vi "Get Temperature Offset.vi"(8 "error in (no error)":errorcluster, 11 "VISA resource name":refnum<visa-resource-name>) -> (0 "error out":errorcluster, 1 "Temperature Units":i32, 2 "Temperature Offset":dbl format="%.4f", 3 "VISA resource name out":refnum<visa-resource-name>)   [LabVIEW 2013, in "Fluke 5XXX Series Multicalibrators.lvlib"]
doc: "This VI returns the temperature offset used for thermocouple measurements (±500 °C).\n\nNote:\n\nThis VI is available only for instrument models 5500A and 5520A."
uses:
  Fluke 5XXX Series Multicalibrators.lvlib
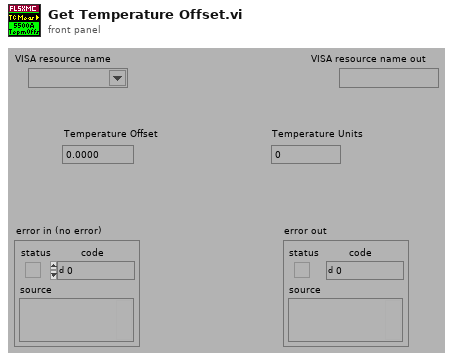
[diagram p1: front panel]
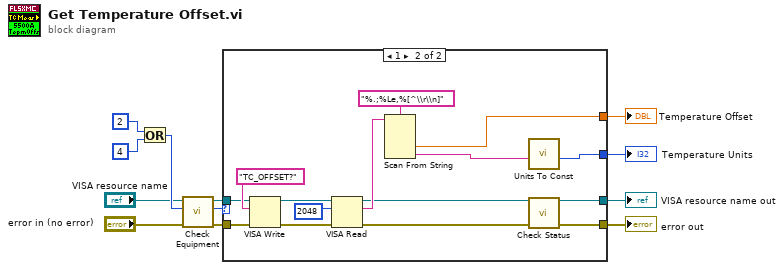
[diagram p0: block diagram]
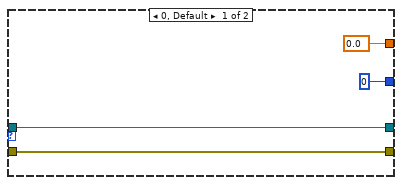
[diagram p2: hidden frame]
diagram:
  n1 = Or(x=2 ("Numeric"), y=4 ("Numeric")) -> (x .or. y?=w8:i32)
  n2 = call "Check Equipment.vi"("error in (no error)"="error in (no error)", "Bit Mask"=w8, "VISA resource name"="VISA resource name") -> ("error out"=w12:errorcluster, "Present?"=w11:u32, "VISA resource name out"=w10:refnum<visa-resource-name>)  [unwired: 6 in]
  n3 = case shown="1" w11 {
    tunnel: [w16 w25] -> w5
    tunnel: [w15 w24] -> w4
    tunnel: w12 -> [w16 w27]
    tunnel: w10 -> [w15 w26]
    tunnel: [0 ("Index") w21] -> w3
    tunnel: [0.0 w17] -> w1
    frame 0, Default {
    }
    frame 1 {
      n4 = VISA Write(VISA resource name=w26, write buffer="TC_OFFSET?", error in (no error)=w27) -> (VISA resource name out=w30:refnum<visa-resource-name>, error out=w29:errorcluster)  [unwired: 1 out]
      n5 = VISA Read(VISA resource name=w30, byte count=u32 2048 ("byte count (0)"), error in (no error)=w29) -> (VISA resource name out=w18:refnum<visa-resource-name>, read buffer=w22:string, error out=w19:errorcluster)  [unwired: 1 out]
      n6 = Scan From String(format string="%.;%Le,%[^\\r\\n]", input string=w22) -> (output 1=w17:dbl, output 2=w20:string)  [unwired: 4 in, 3 out]
      n7 = call "Units To Const.vi"("Units"=w20) -> ("Const"=w21:i32)  [unwired: 10 in]
      n8 = call "Check Status.vi"("VISA resource name"=w18, "error in (no error)"=w19) -> ("VISA resource name out"=w24:refnum<visa-resource-name>, "error out"=w25:errorcluster)  [unwired: 12 in]
    }
  }
  "Temperature Offset" <- w1
  "Temperature Units" <- w3
  "VISA resource name out" <- w4
  "error out" <- w5
